vi "Savitsky Golay Filter (single).vi"(6 "Side Points Unit (points)":enum16{"Points", "Data"}(ring), 8 "error in (no error)":errorcluster, 9 "polynomial order (3)":i32=3, 10 "side points (6)":dbl=6.0, 11 "XY-data":cluster{"X-array":dbl[], "Y-array":dbl[]}) -> (0 "error out":errorcluster, 3 "XY-data out":cluster{"X-array":dbl[], "Y-array":dbl[]} {"Y-array" format="%.2p"; "X-array" format="%.2p"})   [LabVIEW 2019, in "xy_utilities.lvlib"]
doc: "Filter <b>XY-data</b>'s Y-Array with a Savitsky-Golay FIR smoothing filter.\n\n<b>side points</b> specifies the number of data points to each side of the current data point to use for the least squares minimization. side points*2 + 1 is the length of the moving window, which must be greater than the polynomial order.\n\n<b>polynomial order</b> specifies the order of the polynomial. \n\nWire data to the data input to determine the polymorphic instance to use or manually select the instance."
uses:
  xy_utilities.lvlib
  <vilib>/Analysis/NI_AALBase.lvlib
  <vilib>/Analysis/3filter.llb/Savitzky-Golay Filter (DBL).vi
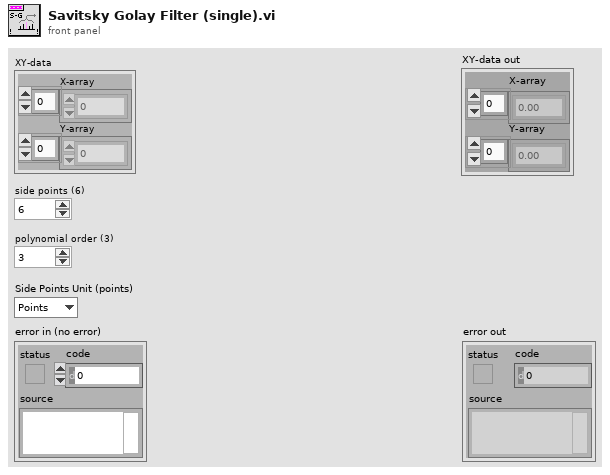
[diagram p1: front panel]
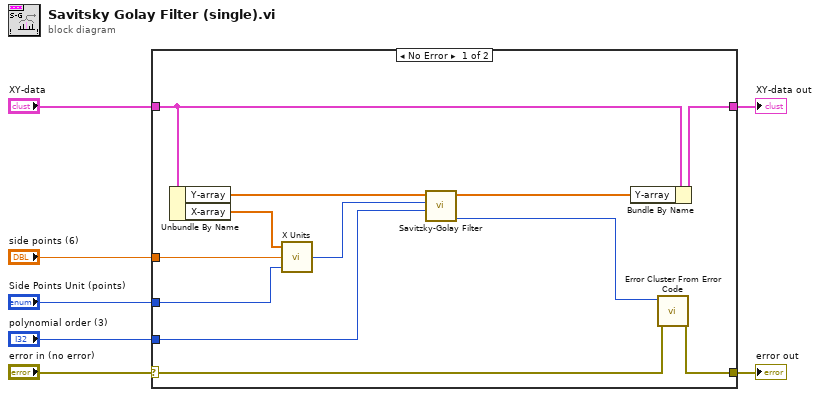
[diagram p0: block diagram]
diagram:
  n1 = case shown="No Error" "error in (no error)" {
    selector: "error in (no error)" -> [w14 w21]
    tunnel: [w13 w21] -> w6
    tunnel: "XY-data" -> [w18 w20]
    tunnel: [w19 w20] -> w4
    tunnel: "side points (6)" -> [w11 _]
    tunnel: "Side Points Unit (points)" -> [w9 _]
    tunnel: "polynomial order (3)" -> [w8 _]
    frame No Error {
      n2 = Unbundle By Name(w18) -> ("Y-array"=w17:dbl[], "X-array"=w12:dbl[])
      n3 = call "X Units.vi"("Interval Units (points)"=w9, "Interval (h)"=w11, "X-array"=w12) -> ("h (points)"=w10:i32)
      n4 = call-poly <vilib>:"Savitzky-Golay Filter.vi"("polynomial order"=w8, "side points"=w10, "X"=w17) -> ("error"=w15:i32, "Filtered X"=w16:dbl[])  [unwired: 7 in]
      n5 = Bundle By Name(cluster=w18, "Y-array"=w16) -> (w19:cluster{"X-array":dbl[], "Y-array":dbl[]})
      n6 = call <vilib>:"Error Cluster From Error Code.vi"("error in (no error)"=w14, "error code (0)"=w15) -> ("error out"=w13:errorcluster)  [unwired: 7 in]
    }
    frame Error {
    }
  }
  "error out" <- w6
  "XY-data out" <- w4
